vi "Generate Fake Vibration Signals.vi"() -> ()   [LabVIEW 2017]
uses:
  <vilib>/DAQmx/write.llb/DAQmx Write (Analog 1D Wfm NChan NSamp).vi
  <vilib>/DAQmx/create/channels.llb/DAQmx Create Channel (AO-Voltage-Basic).vi
  <vilib>/DAQmx/miscellaneous.llb/DAQmx Fill In Error Info.vi
  <resource>/objmgr/daqmx.rc
panel:
  in  "physical channels":tag="Dev2/ao8:31"
  out "Vib System 3":waveform(dbl)[](graph)
  out "Vib System 2":waveform(dbl)[](graph)
  in  "Constant Amplitudes?":bool
  in  "stop":bool
  out "Vib System 1":waveform(dbl)[](graph)
  in  "sampling info":cluster{"Fs":dbl, "#s":dbl}={"Fs"=10000.0, "#s"=10000.0} {"Fs" format="%.2p"}
  in  "Frequency":dbl=60.0 format="%0.2p"
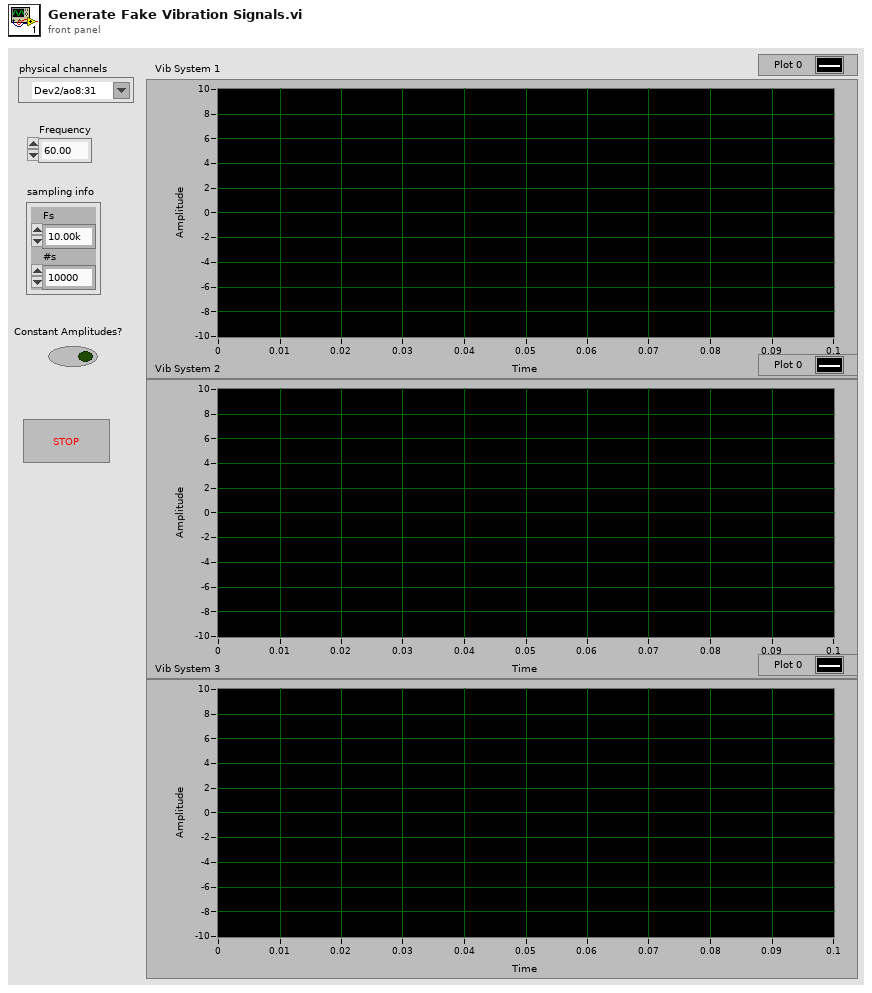
[diagram p1: front panel]
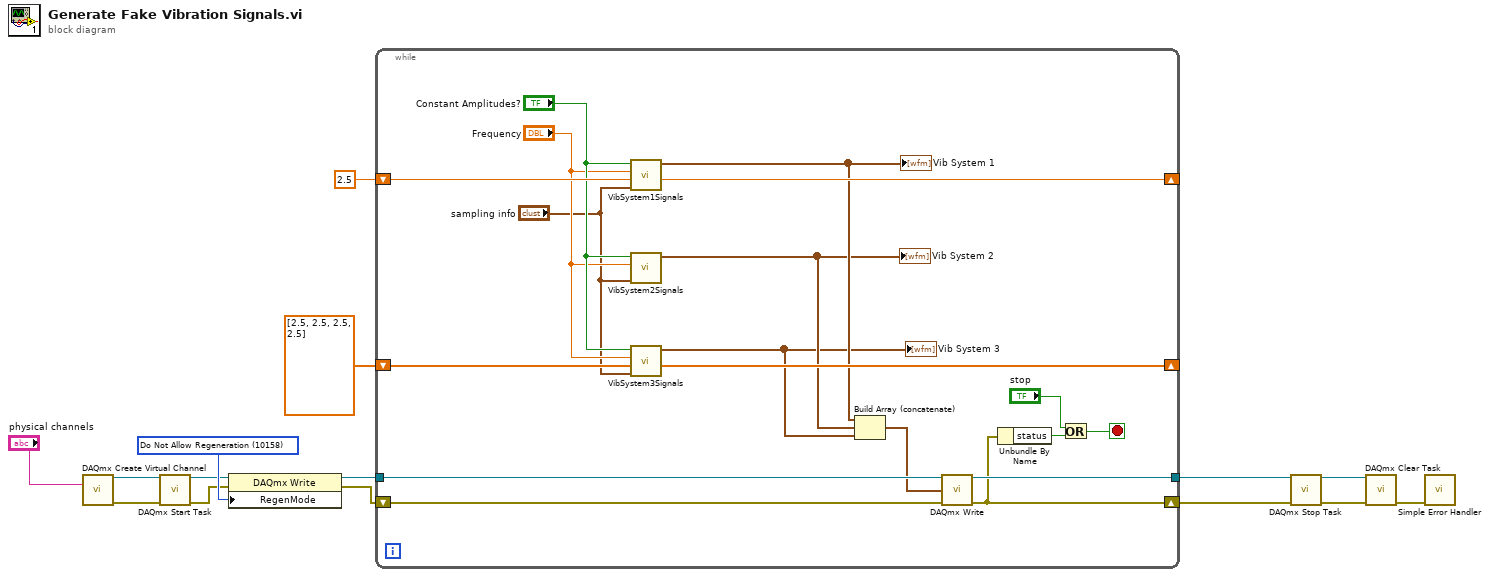
[diagram p0: block diagram]
diagram:
  w5 = 10158 items=["Allow Regeneration"=10097, "Do Not Allow Regeneration"=10158] ("RegenMode")
  n1 = call-poly <vilib>:"DAQmx Create Virtual Channel.vi"("physical channels"="physical channels") -> ("task out"=w13:refnum<k21>, "error out"=w12:errorcluster)  [unwired: 13 in]
  n2 = call <vilib>:"DAQmx Start Task.vi"("task/channels in"=w13, "error in"=w12) -> ("task out"=w4:refnum<k21>, "error out"=w2:errorcluster)  [unwired: 12 in]
  n3 = property class="DAQmx Write"(reference=w4, error in=w2, "RegenMode"=w5) -> (reference out=w3:refnum<k21>, error out=w1:errorcluster)
  n4 = while {
    shift-right: [w32] -> _
    shift-left: 2.5 ("y") -> [w33]
    shift-right: [w28] -> _
    shift-left: dbl[] [2.5, 2.5, 2.5, 2.5] -> [w29]
    tunnel: w3 -> [w26]
    tunnel: [w25] -> w11
    shift-right: [w21] -> w8
    shift-left: w1 -> [w24]
    stop <- w23 stop-if-true
    n5 = call <vilib>:"VibSystem1Signals.vi"("sampling info"="sampling info", "Temperature Channel Voltage In"=w33, "Frequency"="Frequency", "Constant Amplitudes?"="Constant Amplitudes?") -> ("Temperature Channel Voltage Out"=w32:dbl, "Signals"=w19:waveform(dbl)[])  [unwired: 6 in]
    "Vib System 1" <- w19
    n6 = call <vilib>:"VibSystem2Signals.vi"("sampling info"="sampling info", "Frequency"="Frequency", "Constant Amplitudes?"="Constant Amplitudes?") -> ("Signals"=w18:waveform(dbl)[])  [unwired: 8 in]
    "Vib System 2" <- w18
    n7 = call <vilib>:"VibSystem3Signals.vi"("sampling info"="sampling info", "Temperature Channels Voltage In"=w29, "Frequency"="Frequency", "Constant Amplitudes?"="Constant Amplitudes?") -> ("Temperature Channels Voltage Out"=w28:dbl[], "Signals"=w17:waveform(dbl)[])  [unwired: 6 in]
    "Vib System 3" <- w17
    n8 = Build Array (concatenate)(w19, w18, w17) -> (w16:waveform(dbl)[])
    n9 = call-poly <vilib>:"DAQmx Write.vi"("task/channels in"=w26, "data"=w16, "error in"=w24) -> ("task out"=w25:refnum<k21>, "error out"=w21:errorcluster)  [unwired: 10 in, 1 out]
    n10 = Unbundle By Name(w21) -> ("status"=w20:bool)
    n11 = Or(x="stop", y=w20) -> (x .or. y?=w23:bool)
  }
  n12 = call <vilib>:"DAQmx Stop Task.vi"("task/channels in"=w11, "error in"=w8) -> ("task out"=w10:refnum<k21>, "error out"=w9:errorcluster)  [unwired: 12 in]
  n13 = call <vilib>:"DAQmx Clear Task.vi"("task in"=w10, "error in"=w9) -> ("error out"=w7:errorcluster)  [unwired: 13 in]
  n14 = call <vilib>:"Simple Error Handler.vi"("error in (no error)"=w7) -> ()  [unwired: 4 in, 5 out]
